vi "单数据解析.vi"(0 "Data1":u8, 1 "Data2":u8, 2 "Data3":u8, 3 "Data4":u8, 4 "Data5":u8, 5 "Data6":u8, 6 "Data7":u8, 7 "Data8":u8, 8 "ID":i32 format="%x", 9 "选项卡数值":enum32{"单体电压", "单体温度", "单体内阻", "单体SOC"}(ring)) -> (20 "位置":i32[](array[numeric]), 22 "数据":dbl[](array[numeric]), 24 "放电均衡":i32[](array[numeric]), 25 "充电均衡":i32[](array[numeric]), 26 "PF":i32, 27 "均衡故障":dbl[](array[numeric]))   [LabVIEW 2013]
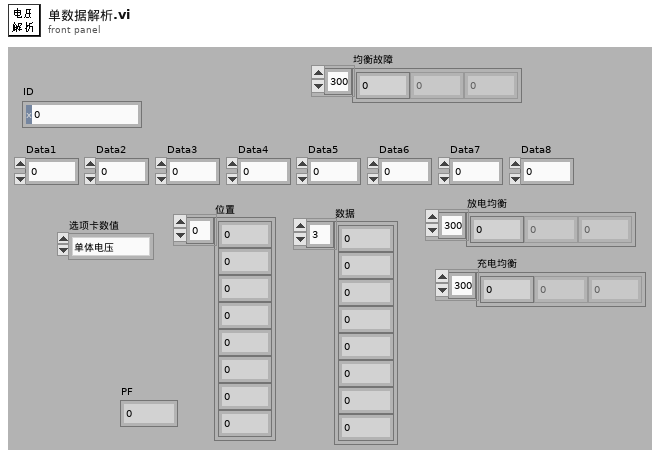
[diagram p1: front panel]
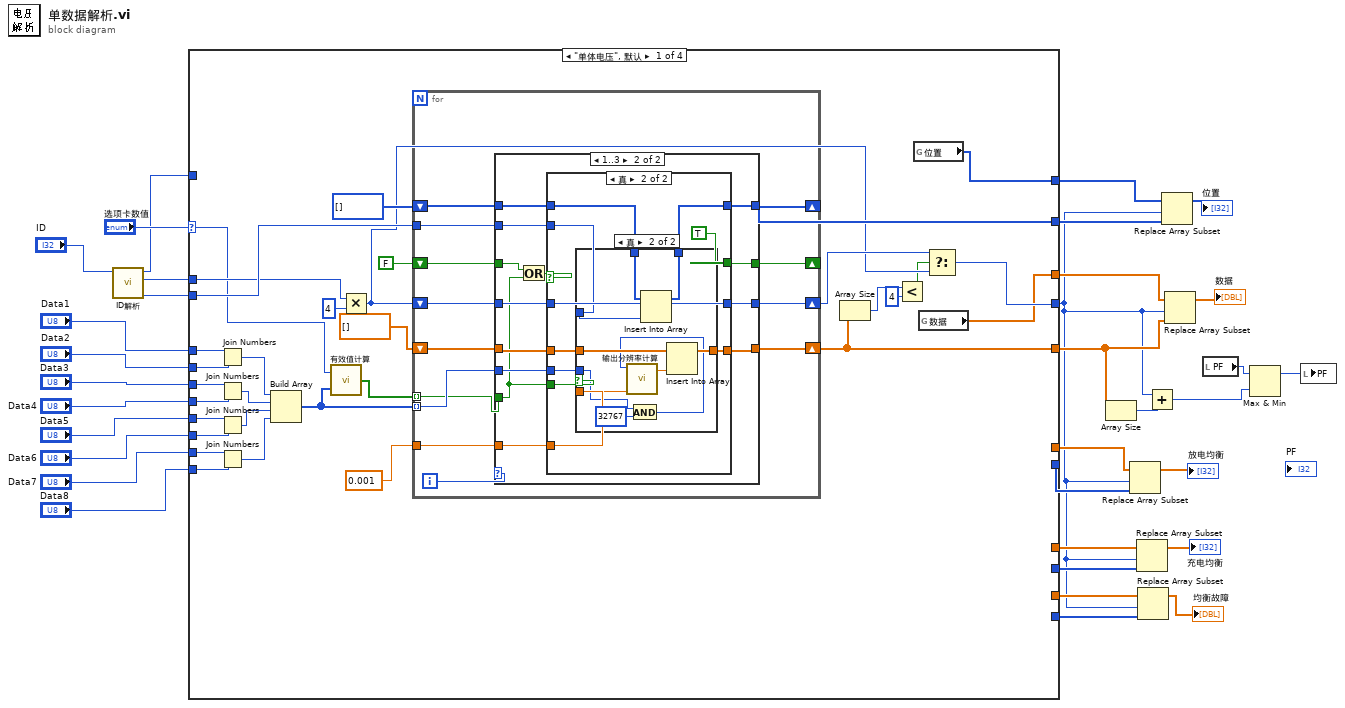
[diagram p0: block diagram]
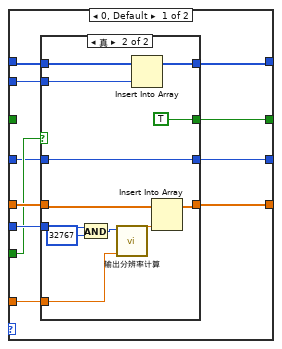
[diagram p2: hidden frame]
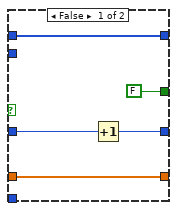
[diagram p3: hidden frame]
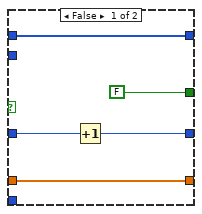
[diagram p4: hidden frame]
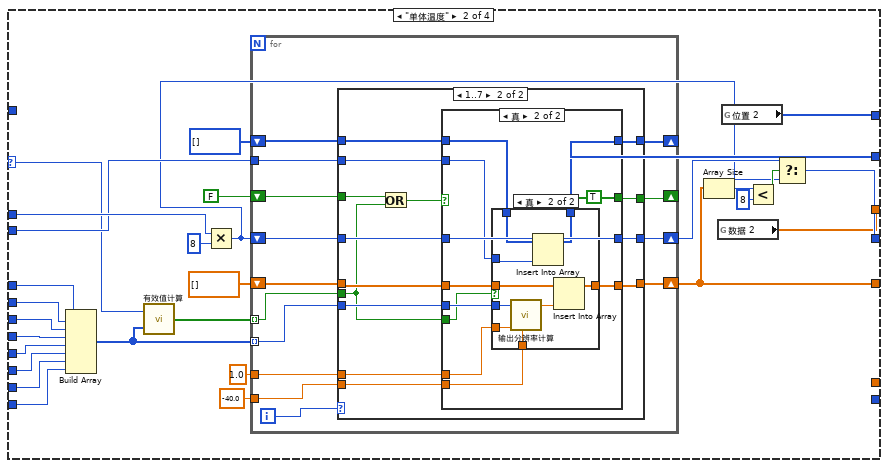
[diagram p6: hidden frame]
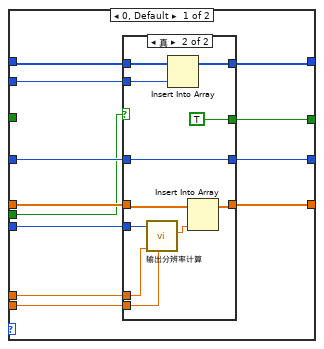
[diagram p7: hidden frame]
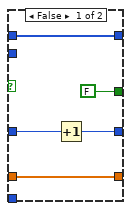
[diagram p8: hidden frame]
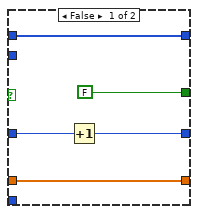
[diagram p9: hidden frame]
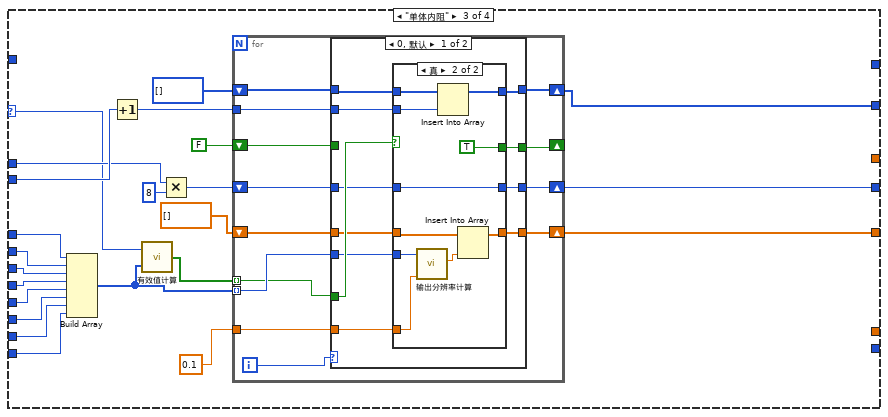
[diagram p11: hidden frame]
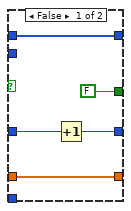
[diagram p12: hidden frame]
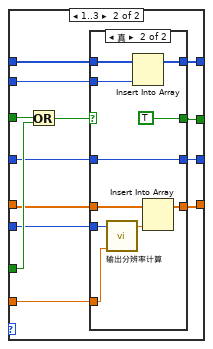
[diagram p13: hidden frame]
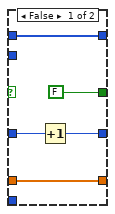
[diagram p14: hidden frame]
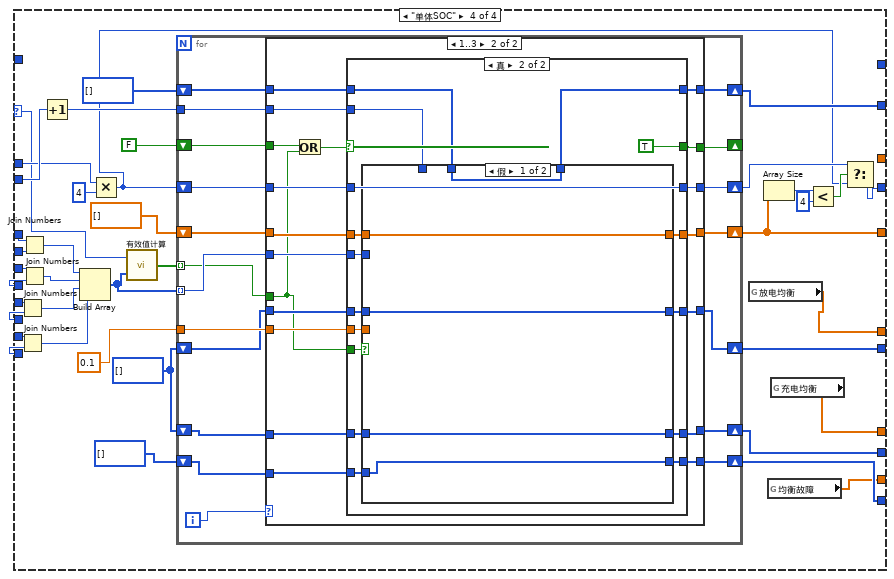
[diagram p15: hidden frame]
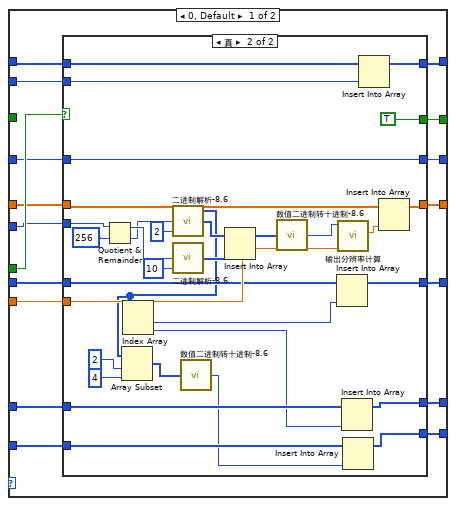
[diagram p16: hidden frame]
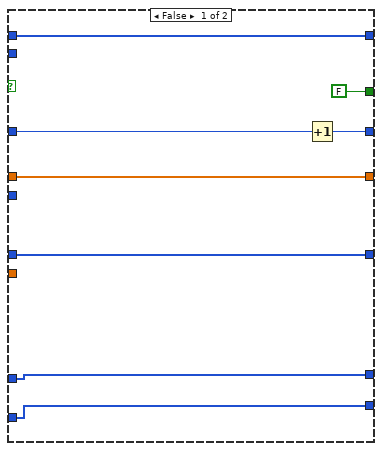
[diagram p17: hidden frame]
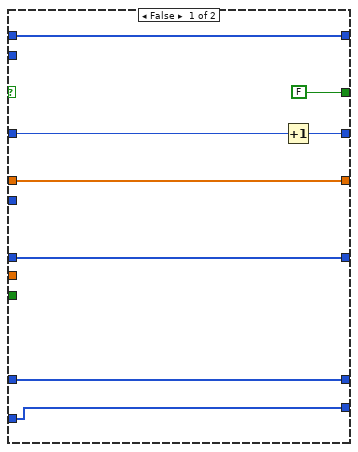
[diagram p18: hidden frame]
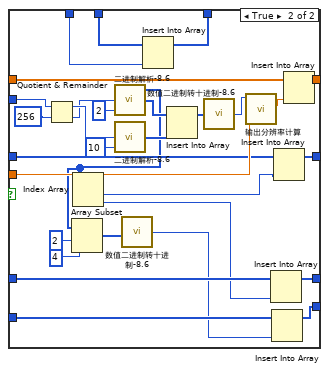
[diagram p19: hidden frame]
diagram:
  n1 = call "ID解析.vi"("ID"="ID") -> ("SA(4)"=w18:i32, "PF(2)"=w17:i32, "PDU(1)"=w29:i32)  [unwired: 8 out]
  n2 = case shown="\"单体电压\", 默认" "选项卡数值" {
    selector: "选项卡数值" -> [w34 w147 w260 w350]
    tunnel: "Data2" -> [w65 w173 w268 w379]
    tunnel: "Data1" -> [w64 w174 w269 w378]
    tunnel: "Data3" -> [w63 w172 w267 w377]
    tunnel: "Data4" -> [w62 w171 w266 w376]
    tunnel: "Data5" -> [w61 w170 w265 w375]
    tunnel: "Data7" -> [w60 w168 w263 w373]
    tunnel: "Data8" -> [w59 w167 w262 w372]
    tunnel: "Data6" -> [w58 w169 w264 w374]
    tunnel: [w56 w164 w278 w356] -> w3
    tunnel: [w57 w175 w273 w381] -> w33
    tunnel: [w55 w166 w272 w360] -> w5
    tunnel: w18 -> [w54 w163 w271 w380]
    tunnel: w17 -> [w53 w165 w270 w358]
    tunnel: [_ _ _ w367] -> w14
    tunnel: w29 -> [_ _ _ _]
    tunnel: [w38 w151 _ _] -> w16
    tunnel: [w37 w150 _ _] -> w15
    tunnel: [_ _ _ w366] -> w13
    tunnel: [_ _ _ w365] -> w12
    tunnel: [_ _ _ w355] -> w9
    tunnel: [_ _ _ w353] -> w8
    tunnel: [_ _ _ w352] -> w7
    frame "单体电压", Default {
      n3 = Join Numbers(hi=w64, lo=w65) -> ((hi.lo)=w51:u16)
      n4 = Join Numbers(hi=w63, lo=w62) -> ((hi.lo)=w50:u16)
      n5 = Join Numbers(hi=w61, lo=w58) -> ((hi.lo)=w49:u16)
      n6 = Join Numbers(hi=w60, lo=w59) -> ((hi.lo)=w48:u16)
      n7 = Build Array(w51, w50, w49, w48) -> (w36:u16[])
      n8 = call "有效值计算.vi"("数组"=w36, "选项卡数值"=w34) -> ("有效位"=w35:bool[])
      n9 = Multiply(x=w53, y=4) -> (x*y=w42:i32)
      n10 = for {
        tunnel: w36 -> [w75] mode=indexing
        shift-right: [w76] -> w55
        shift-left: dbl[] [] -> [w77]
        tunnel: 0.001 ("分辨率") -> [w74]
        shift-right: [w72] -> w57
        shift-left: i32[] [] -> [w73]
        tunnel: w54 -> [w71]
        shift-right: [w70] -> _
        shift-left: FALSE -> [w69]
        shift-right: [w67] -> w43
        shift-left: w42 -> [w68]
        tunnel: w35 -> [w66] mode=indexing
        i -> [w78]
        n11 = case shown="1..3" w78 {
          tunnel: w66 -> [w81 w107]
          tunnel: [w89 w119] -> w70
          tunnel: w77 -> [w88 w118]
          tunnel: [w87 w117] -> w76
          tunnel: w75 -> [w86 w116]
          tunnel: w74 -> [w85 w115]
          tunnel: w73 -> [w84 w114]
          tunnel: [w83 w113] -> w72
          tunnel: w71 -> [w82 w112]
          tunnel: w69 -> [_ w108]
          tunnel: w68 -> [w80 w111]
          tunnel: [w79 w110] -> w67
          frame 0, Default {
            n12 = case shown="真" w81 {
              tunnel: [FALSE TRUE] -> w89
              tunnel: w88 -> [w93 w105]
              tunnel: [w93 w104] -> w87
              tunnel: w86 -> [_ w97]
              tunnel: w85 -> [_ w102]
              tunnel: w84 -> [w92 w101]
              tunnel: [w92 w100] -> w83
              tunnel: w82 -> [_ w99]
              tunnel: w80 -> [w91 w98]
              tunnel: [w90 w98] -> w79
              frame False {
                n13 = Increment(x=w91) -> (x+1=w90:i32)
              }
              frame True {
                n14 = And(x=w97, y=u16 32767) -> (x .and. y?=w95:u16)
                n15 = call "输出分辨率计算.vi"("分辨率"=w102, "数值 2"=w95) -> ("输出2"=w103:dbl)  [unwired: 4 in, 5 out]
                n16 = Insert Into Array(array=w101, new element=w99) -> (w100:i32[])  [unwired: 1 in]
                n17 = Insert Into Array(array=w105, new element=w103) -> (w104:dbl[])  [unwired: 1 in]
              }
            }
          }
          frame 1..3 {
            n18 = Or(x=w108, y=w107) -> (x .or. y?=w109:bool)
            n19 = case shown="真" w109 {
              tunnel: [FALSE TRUE] -> w119
              tunnel: w118 -> [w124 w133]
              tunnel: [w124 w132] -> w117
              tunnel: w116 -> [_ w131]
              tunnel: w115 -> [_ w130]
              tunnel: w114 -> [w123 w126]
              tunnel: [w123 w125] -> w113
              tunnel: w112 -> [_ w127]
              tunnel: w111 -> [w121 w129]
              tunnel: [w120 w129] -> w110
              tunnel: w107 -> [_ w128]
              frame False {
                n20 = Increment(x=w121) -> (x+1=w120:i32)
              }
              frame True {
                n21 = case shown="真" w128 {
                  tunnel: w133 -> [w136 w146]
                  tunnel: [w136 w145] -> w132
                  tunnel: w131 -> [_ w138]
                  tunnel: w130 -> [_ w144]
                  tunnel: w127 -> [_ w142]
                  tunnel: w126 -> [w135 w141]
                  tunnel: [w135 w140] -> w125
                  frame False {
                  }
                  frame True {
                    n22 = And(x=w138, y=u16 32767) -> (x .and. y?=w137:u16)
                    n23 = call "输出分辨率计算.vi"("分辨率"=w144, "数值 2"=w137) -> ("输出2"=w143:dbl)  [unwired: 4 in, 5 out]
                    n24 = Insert Into Array(array=w141, new element=w142) -> (w140:i32[])  [unwired: 1 in]
                    n25 = Insert Into Array(array=w146, new element=w143) -> (w145:dbl[])  [unwired: 1 in]
                  }
                }
              }
            }
          }
        }
      }
      n26 = Array Size(array=w55) -> (size(s)=w41:i32)
      n27 = Less?(x=w41, y=4) -> (x < y?=w39:bool)
      n28 = global read "单体信息全局.vi" "位置"() -> (w38:i32[])
      n29 = global read "单体信息全局.vi" "数据"() -> (w37:dbl[])
      n30 = Select(t=w43, s=w39, f=w42) -> (s? t:f=w56:i32)
    }
    frame "单体温度" {
      n31 = Build Array(w174, w173, w172, w171, w170, w169, w168, w167) -> (w149:u8[])
      n32 = call "有效值计算.vi"("数组"=w149, "选项卡数值"=w147) -> ("有效位"=w148:bool[])
      n33 = Multiply(x=w165, y=8) -> (x*y=w152:i32)
      n34 = for {
        tunnel: w149 -> [w182] mode=indexing
        shift-right: [w187] -> w153
        shift-left: w152 -> [w188]
        shift-right: [w186] -> _
        shift-left: FALSE -> [w185]
        shift-right: [w183] -> w166
        shift-left: dbl[] [] -> [w184]
        tunnel: 1.0 ("分辨率") -> [w181]
        shift-right: [w179] -> w175
        shift-left: i32[] [] -> [w180]
        tunnel: w163 -> [w178]
        tunnel: -40.0 ("分辨率") -> [w177]
        tunnel: w148 -> [w176] mode=indexing
        i -> [w189]
        n35 = case shown="1..7" w189 {
          tunnel: w188 -> [w201 w229]
          tunnel: [w200 w228] -> w187
          tunnel: [w199 w227] -> w186
          tunnel: w185 -> [_ w230]
          tunnel: w184 -> [w198 w226]
          tunnel: [w197 w225] -> w183
          tunnel: w182 -> [w196 w224]
          tunnel: w181 -> [w195 w223]
          tunnel: w180 -> [w194 w222]
          tunnel: [w193 w221] -> w179
          tunnel: w178 -> [w192 w220]
          tunnel: w177 -> [w191 w219]
          tunnel: w176 -> [w190 w218]
          frame 0, Default {
            n36 = case shown="真" w190 {
              tunnel: w201 -> [w205 w217]
              tunnel: [w204 w217] -> w200
              tunnel: [FALSE TRUE] -> w199
              tunnel: w198 -> [w203 w215]
              tunnel: [w203 w214] -> w197
              tunnel: w196 -> [_ w213]
              tunnel: w195 -> [_ w211]
              tunnel: w194 -> [w202 w210]
              tunnel: [w202 w209] -> w193
              tunnel: w192 -> [_ w208]
              tunnel: w191 -> [_ w207]
              frame False {
                n37 = Increment(x=w205) -> (x+1=w204:i32)
              }
              frame True {
                n38 = call "输出分辨率计算.vi"("偏移量"=w207, "分辨率"=w211, "数值 2"=w213) -> ("输出2"=w212:dbl)  [unwired: 3 in, 5 out]
                n39 = Insert Into Array(array=w210, new element=w208) -> (w209:i32[])  [unwired: 1 in]
                n40 = Insert Into Array(array=w215, new element=w212) -> (w214:dbl[])  [unwired: 1 in]
              }
            }
          }
          frame 1..7 {
            n41 = Or(x=w230, y=w218) -> (x .or. y?=w231:bool)
            n42 = case shown="真" w231 {
              tunnel: w229 -> [w236 w247]
              tunnel: [w235 w247] -> w228
              tunnel: [FALSE TRUE] -> w227
              tunnel: w226 -> [w233 w245]
              tunnel: [w233 w244] -> w225
              tunnel: w224 -> [_ w243]
              tunnel: w223 -> [_ w242]
              tunnel: w222 -> [w232 w239]
              tunnel: [w232 w238] -> w221
              tunnel: w220 -> [_ w240]
              tunnel: w219 -> [_ w241]
              tunnel: w218 -> [_ w237]
              frame False {
                n43 = Increment(x=w236) -> (x+1=w235:i32)
              }
              frame True {
                n44 = case shown="真" w237 {
                  tunnel: w245 -> [w249 w258]
                  tunnel: [w249 w257] -> w244
                  tunnel: w243 -> [_ w256]
                  tunnel: w242 -> [_ w255]
                  tunnel: w241 -> [_ w254]
                  tunnel: w240 -> [_ w252]
                  tunnel: w239 -> [w248 w251]
                  tunnel: [w248 w250] -> w238
                  frame False {
                  }
                  frame True {
                    n45 = call "输出分辨率计算.vi"("偏移量"=w254, "分辨率"=w255, "数值 2"=w256) -> ("输出2"=w253:dbl)  [unwired: 3 in, 5 out]
                    n46 = Insert Into Array(array=w251, new element=w252) -> (w250:i32[])  [unwired: 1 in]
                    n47 = Insert Into Array(array=w258, new element=w253) -> (w257:dbl[])  [unwired: 1 in]
                  }
                }
              }
            }
          }
        }
      }
      n48 = Array Size(array=w166) -> (size(s)=w156:i32)
      n49 = global read "单体信息全局.vi" "数据 2"() -> (w150:dbl[])
      n50 = global read "单体信息全局.vi" "位置 2"() -> (w151:i32[])
      n51 = Less?(x=w156, y=8) -> (x < y?=w154:bool)
      n52 = Select(t=w153, s=w154, f=w152) -> (s? t:f=w164:i32)
    }
    frame "单体内阻" {
      n53 = Build Array(w269, w268, w267, w266, w265, w264, w263, w262) -> (w261:u8[])
      n54 = Increment(x=w271) -> (x+1=w275:i32)
      n55 = call "有效值计算.vi"("数组"=w261, "选项卡数值"=w260) -> ("有效位"=w259:bool[])
      n56 = Multiply(x=w270, y=8) -> (x*y=w280:i32)
      n57 = for {
        tunnel: w261 -> [w287] mode=indexing
        shift-right: [w292] -> w278
        shift-left: w280 -> [w293]
        shift-right: [w291] -> _
        shift-left: FALSE -> [w290]
        shift-right: [w288] -> w272
        shift-left: dbl[] [] -> [w289]
        tunnel: 0.1 ("分辨率") -> [w286]
        shift-right: [w284] -> w273
        shift-left: i32[] [] -> [w285]
        tunnel: w275 -> [w283]
        tunnel: w259 -> [w282] mode=indexing
        i -> [w294]
        n58 = case shown="0, 默认" w294 {
          tunnel: w282 -> [w305 w331]
          tunnel: w293 -> [w304 w330]
          tunnel: [w303 w329] -> w292
          tunnel: [w302 w328] -> w291
          tunnel: w290 -> [_ w332]
          tunnel: w289 -> [w301 w327]
          tunnel: [w300 w326] -> w288
          tunnel: w287 -> [w299 w325]
          tunnel: w286 -> [w298 w324]
          tunnel: w285 -> [w297 w323]
          tunnel: [w296 w322] -> w284
          tunnel: w283 -> [w295 w321]
          frame 0, Default {
            n59 = case shown="真" w305 {
              tunnel: w304 -> [w309 w320]
              tunnel: [w308 w320] -> w303
              tunnel: [FALSE TRUE] -> w302
              tunnel: w301 -> [w307 w318]
              tunnel: [w307 w317] -> w300
              tunnel: w299 -> [_ w316]
              tunnel: w298 -> [_ w314]
              tunnel: w297 -> [w306 w313]
              tunnel: [w306 w312] -> w296
              tunnel: w295 -> [_ w311]
              frame False {
                n60 = Increment(x=w309) -> (x+1=w308:i32)
              }
              frame True {
                n61 = call "输出分辨率计算.vi"("分辨率"=w314, "数值 2"=w316) -> ("输出2"=w315:dbl)  [unwired: 4 in, 5 out]
                n62 = Insert Into Array(array=w313, new element=w311) -> (w312:i32[])  [unwired: 1 in]
                n63 = Insert Into Array(array=w318, new element=w315) -> (w317:dbl[])  [unwired: 1 in]
              }
            }
          }
          frame 1..3 {
            n64 = Or(x=w332, y=w331) -> (x .or. y?=w333:bool)
            n65 = case shown="真" w333 {
              tunnel: w330 -> [w338 w348]
              tunnel: [w337 w348] -> w329
              tunnel: [FALSE TRUE] -> w328
              tunnel: w327 -> [w335 w346]
              tunnel: [w335 w345] -> w326
              tunnel: w325 -> [_ w344]
              tunnel: w324 -> [_ w342]
              tunnel: w323 -> [w334 w341]
              tunnel: [w334 w340] -> w322
              tunnel: w321 -> [_ w339]
              frame False {
                n66 = Increment(x=w338) -> (x+1=w337:i32)
              }
              frame True {
                n67 = call "输出分辨率计算.vi"("分辨率"=w342, "数值 2"=w344) -> ("输出2"=w343:dbl)  [unwired: 4 in, 5 out]
                n68 = Insert Into Array(array=w341, new element=w339) -> (w340:i32[])  [unwired: 1 in]
                n69 = Insert Into Array(array=w346, new element=w343) -> (w345:dbl[])  [unwired: 1 in]
              }
            }
          }
        }
      }
    }
    frame "单体SOC" {
      w364 = i32[] []
      n70 = Join Numbers(hi=w375, lo=w374) -> ((hi.lo)=w370:u16)
      n71 = Join Numbers(hi=w373, lo=w372) -> ((hi.lo)=w371:u16)
      n72 = Join Numbers(hi=w378, lo=w379) -> ((hi.lo)=w368:u16)
      n73 = Join Numbers(hi=w377, lo=w376) -> ((hi.lo)=w369:u16)
      n74 = Increment(x=w380) -> (x+1=w383:i32)
      n75 = Build Array(w368, w369, w370, w371) -> (w351:u16[])
      n76 = Multiply(x=w358, y=4) -> (x*y=w357:i32)
      n77 = call "有效值计算.vi"("数组"=w351, "选项卡数值"=w350) -> ("有效位"=w349:bool[])
      n78 = for {
        tunnel: w351 -> [w393] mode=indexing
        shift-right: [w404] -> w359
        shift-left: w357 -> [w405]
        shift-right: [w403] -> _
        shift-left: FALSE -> [w402]
        shift-right: [w400] -> w360
        shift-left: dbl[] [] -> [w401]
        tunnel: 0.1 ("分辨率") -> [w399]
        shift-right: [w397] -> w381
        shift-left: i32[] [] -> [w398]
        tunnel: w383 -> [w396]
        shift-right: [w394] -> w367
        shift-left: w364 -> [w395]
        shift-right: [w391] -> w355
        shift-left: w364 -> [w392]
        shift-right: [w389] -> w353
        shift-left: i32[] [] -> [w390]
        tunnel: w349 -> [w388] mode=indexing
        i -> [w406]
        n79 = case shown="1..3" w406 {
          tunnel: w388 -> [w423 w464]
          tunnel: w405 -> [w422 w480]
          tunnel: [w421 w479] -> w404
          tunnel: [w420 w478] -> w403
          tunnel: w402 -> [_ w481]
          tunnel: w401 -> [w419 w477]
          tunnel: [w418 w476] -> w400
          tunnel: w393 -> [w411 w475]
          tunnel: w399 -> [w417 w474]
          tunnel: w398 -> [w416 w473]
          tunnel: [w415 w472] -> w397
          tunnel: w396 -> [w414 w471]
          tunnel: [w413 w469] -> w394
          tunnel: w395 -> [w412 w470]
          tunnel: w392 -> [w410 w468]
          tunnel: [w409 w467] -> w391
          tunnel: w390 -> [w408 w466]
          tunnel: [w407 w465] -> w389
          frame 0, Default {
            n80 = case shown="真" w423 {
              tunnel: w422 -> [w430 w463]
              tunnel: [w429 w463] -> w421
              tunnel: [FALSE TRUE] -> w420
              tunnel: w419 -> [w428 w461]
              tunnel: [w428 w460] -> w418
              tunnel: w417 -> [_ w458]
              tunnel: w416 -> [w427 w457]
              tunnel: [w427 w456] -> w415
              tunnel: w414 -> [_ w455]
              tunnel: [w426 w454] -> w413
              tunnel: w412 -> [w426 w453]
              tunnel: w411 -> [_ w445]
              tunnel: w410 -> [w425 w443]
              tunnel: [w425 w442] -> w409
              tunnel: w408 -> [w424 w435]
              tunnel: [w424 w434] -> w407
              frame False {
                n81 = Increment(x=w430) -> (x+1=w429:i32)
              }
              frame True {
                n82 = Quotient & Remainder(x=w445, y=u16 256) -> (x-y*floor(x/y)=w451:u16, floor(x/y)=w450:u16)
                n83 = call "二进制解析-8.6.vi"("索引"=2, "数值"=w450) -> ("低位子数组"=w448:i32[], "高位子数组"=w438:i32[])  [unwired: 2 out]
                n84 = Array Subset(array=w438, index=2 ("索引"), length=4 ("长度")) -> (w433:i32[])
                n85 = Index Array(array=w438) -> (element #1=w441:i32, element #2=w440:i32)  [unwired: 2 in]
                n86 = call "二进制解析-8.6.vi"("索引"=10, "数值"=w451) -> ("低位子数组"=w447:i32[])  [unwired: 3 out]
                n87 = call "数值二进制转十进制-8.6.vi"("子数组"=w433) -> ("十进制数值"=w432:i32)  [unwired: 4 out]
                n88 = Insert Into Array(array=w448, new element=w447) -> (w446:i32[])  [unwired: 1 in]
                n89 = call "数值二进制转十进制-8.6.vi"("子数组"=w446) -> ("十进制数值"=w444:i32)  [unwired: 4 out]
                n90 = Insert Into Array(array=w453, new element=w441) -> (w454:i32[])  [unwired: 1 in]
                n91 = call "输出分辨率计算.vi"("分辨率"=w458, "数值 2"=w444) -> ("输出2"=w459:dbl)  [unwired: 4 in, 5 out]
                n92 = Insert Into Array(array=w443, new element=w440) -> (w442:i32[])  [unwired: 1 in]
                n93 = Insert Into Array(array=w435, new element=w432) -> (w434:i32[])  [unwired: 1 in]
                n94 = Insert Into Array(array=w457, new element=w455) -> (w456:i32[])  [unwired: 1 in]
                n95 = Insert Into Array(array=w461, new element=w459) -> (w460:dbl[])  [unwired: 1 in]
              }
            }
          }
          frame 1..3 {
            n96 = Or(x=w481, y=w464) -> (x .or. y?=w482:bool)
            n97 = case shown="真" w482 {
              tunnel: w480 -> [w490 w506]
              tunnel: [w489 w506] -> w479
              tunnel: [FALSE TRUE] -> w478
              tunnel: w477 -> [w487 w504]
              tunnel: [w487 w503] -> w476
              tunnel: w475 -> [_ w499]
              tunnel: w474 -> [_ w502]
              tunnel: w473 -> [w486 w493]
              tunnel: [w486 w491] -> w472
              tunnel: w471 -> [_ w492]
              tunnel: w470 -> [w485 w501]
              tunnel: [w485 w500] -> w469
              tunnel: w468 -> [w484 w498]
              tunnel: [w484 w497] -> w467
              tunnel: w466 -> [w483 w496]
              tunnel: [w483 w495] -> w465
              tunnel: w464 -> [_ w494]
              frame False {
                n98 = Increment(x=w490) -> (x+1=w489:i32)
              }
              frame True {
                n99 = case shown="假" w494 {
                  tunnel: w504 -> [w511 w541]
                  tunnel: [w511 w540] -> w503
                  tunnel: w502 -> [_ w539]
                  tunnel: w501 -> [w510 w538]
                  tunnel: [w510 w537] -> w500
                  tunnel: w499 -> [_ w536]
                  tunnel: w498 -> [w509 w535]
                  tunnel: [w509 w534] -> w497
                  tunnel: w496 -> [w508 w533]
                  tunnel: [w508 w532] -> w495
                  tunnel: w493 -> [w507 w514]
                  tunnel: w492 -> [_ w513]
                  tunnel: [w507 w512] -> w491
                  frame False {
                  }
                  frame True {
                    n100 = Quotient & Remainder(x=w536, y=u16 256) -> (x-y*floor(x/y)=w528:u16, floor(x/y)=w527:u16)
                    n101 = call "二进制解析-8.6.vi"("索引"=2, "数值"=w527) -> ("低位子数组"=w525:i32[], "高位子数组"=w520:i32[])  [unwired: 2 out]
                    n102 = Array Subset(array=w520, index=2 ("索引"), length=4 ("长度")) -> (w516:i32[])
                    n103 = Index Array(array=w520) -> (element #1=w519:i32, element #2=w521:i32)  [unwired: 2 in]
                    n104 = call "二进制解析-8.6.vi"("索引"=10, "数值"=w528) -> ("低位子数组"=w524:i32[])  [unwired: 3 out]
                    n105 = call "数值二进制转十进制-8.6.vi"("子数组"=w516) -> ("十进制数值"=w515:i32)  [unwired: 4 out]
                    n106 = Insert Into Array(array=w514, new element=w513) -> (w512:i32[])  [unwired: 1 in]
                    n107 = Insert Into Array(array=w525, new element=w524) -> (w523:i32[])  [unwired: 1 in]
                    n108 = call "数值二进制转十进制-8.6.vi"("子数组"=w523) -> ("十进制数值"=w522:i32)  [unwired: 4 out]
                    n109 = call "输出分辨率计算.vi"("分辨率"=w539, "数值 2"=w522) -> ("输出2"=w531:dbl)  [unwired: 4 in, 5 out]
                    n110 = Insert Into Array(array=w535, new element=w521) -> (w534:i32[])  [unwired: 1 in]
                    n111 = Insert Into Array(array=w533, new element=w515) -> (w532:i32[])  [unwired: 1 in]
                    n112 = Insert Into Array(array=w538, new element=w519) -> (w537:i32[])  [unwired: 1 in]
                    n113 = Insert Into Array(array=w541, new element=w531) -> (w540:dbl[])  [unwired: 1 in]
                  }
                }
              }
            }
          }
        }
      }
      n114 = global read "单体信息全局.vi" "放电均衡"() -> (w366:dbl[])
      n115 = Array Size(array=w360) -> (size(s)=w363:i32)
      n116 = global read "单体信息全局.vi" "均衡故障"() -> (w352:dbl[])
      n117 = global read "单体信息全局.vi" "充电均衡"() -> (w365:dbl[])
      n118 = Less?(x=w363, y=4) -> (x < y?=w361:bool)
      n119 = Select(t=w359, s=w361, f=w357) -> (s? t:f=w356:i32)
    }
  }
  n120 = Array Size(array=w5) -> (size(s)=w4:i32)
  n121 = Replace Array Subset(array=w13, new element=w14, index=w3) -> (→"放电均衡":dbl[])
  n122 = Replace Array Subset(array=w12, new element=w9, index=w3) -> (→"充电均衡":dbl[])
  n123 = Replace Array Subset(array=w7, new element=w8, index=w3) -> (→"均衡故障":dbl[])
  n124 = Add(x=w3, y=w4) -> (x+y=w2:i32)
  n125 = Replace Array Subset(array=w16, new element=w33, index=w3) -> (→"位置":i32[])
  n126 = Replace Array Subset(array=w15, new element=w5, index=w3) -> (→"数据":dbl[])
  n127 = local read "PF"() -> (w28:i32)
  n128 = Max & Min(x=w28, y=w2) -> (max(x,y)=w1:i32)  [unwired: 1 out]
  n129 = local write "PF"(w1) -> ()
